vi "Read Frequency.vi"(11 "IMD in":refnum<class "IMD.lvclass">) -> (2 "Frequency":cluster{"List":dbl[], "Index":i32, "Last":bool}, 3 "IMD out":refnum<class "IMD.lvclass">)   [LabVIEW 2020, in "IMD.lvclass"]
uses:
  IMD.lvclass
  IMD.lvclass/IMD.ctl
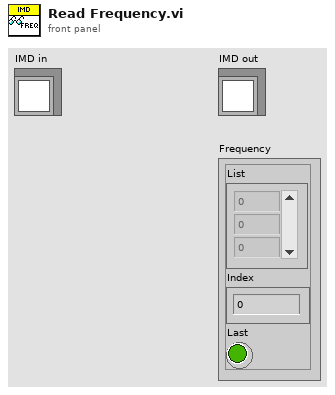
[diagram p1: front panel]
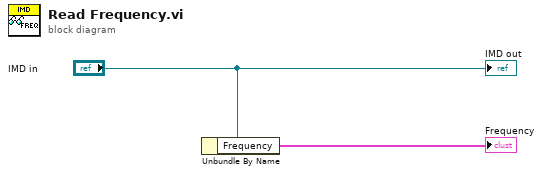
[diagram p0: block diagram]
diagram:
  n1 = Unbundle By Name("IMD in") -> ("Frequency"=→"Frequency":cluster{"List":dbl[], "Index":i32, "Last":bool})
  "IMD out" <- "IMD in"
